vi "Twitter Open.vi"(4 "Access Token Secret (In)":string, 6 "Access Token (In)":string, 8 "error in":errorcluster, 10 "Consumer Secret":string, 11 "Consumer Key":string) -> (0 "error out":errorcluster, 1 "Access Token Secret (Out)":string, 2 "Access Token (Out)":string, 3 "Twitter Handle Out":T1={"OAuth Credentials"={"Signature Method"=enum."HMAC-SHA1", "Version"="1.0", "Client"={"Token"="", "Secret"=""}, "Access"={"Token"="", "Secret"=""}}, "since ID"="", "max ID"="", "Screen Name"=""})   [LabVIEW 2011, in "i3-twitter.lvlib"]
uses:
  i3-twitter.lvlib
  Controls/Twitter Handle.ctl
  i3-oauth/Controls/OAuth Handle.ctl
  i3-oauth/Controls/Signature Method.ctl
  i3-oauth/Controls/Credentials.ctl
  i3-oauth/Controls/Authorization URLs.ctl
  i3-oauth/i3-oauth.lvlib
panel:
  out "Response Header":string
  out "Response Body":string
  # "Debug Only"
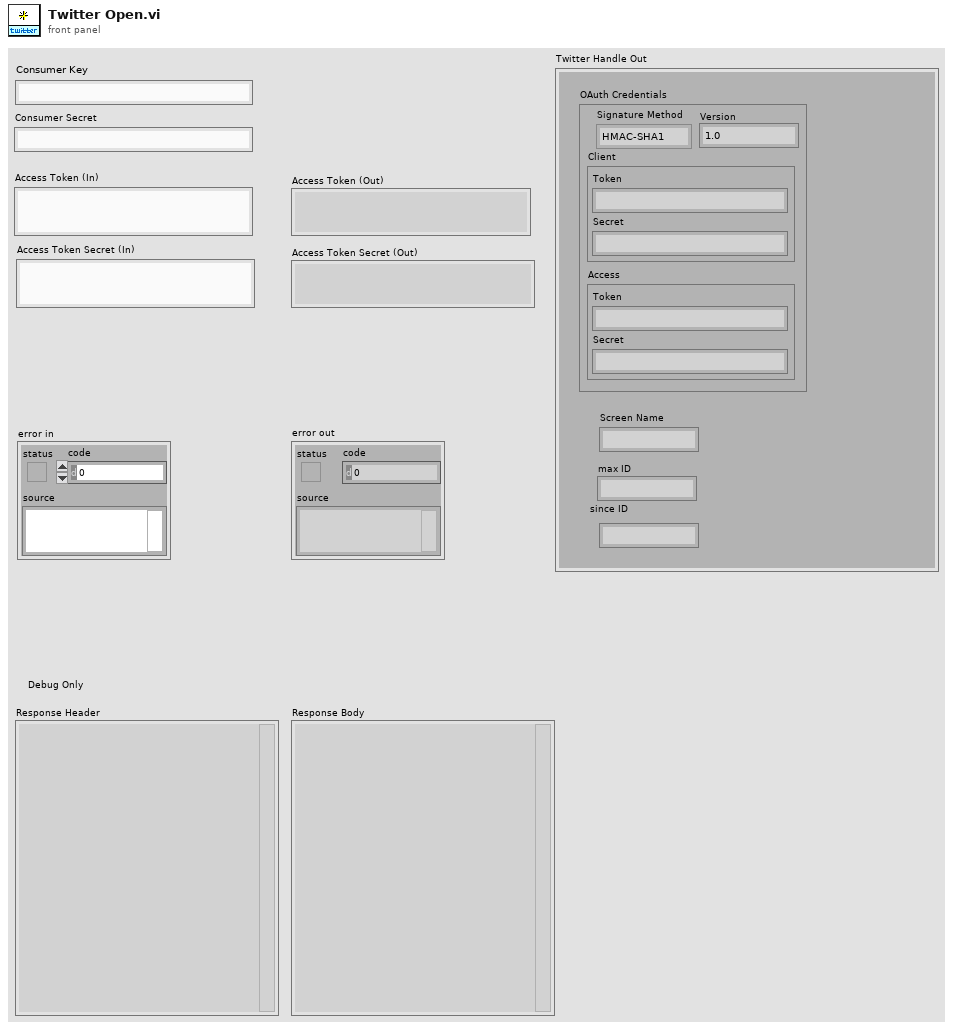
[diagram p1: front panel]
types:
  T1 = typedef "i3-twitter.lvlib/Twitter Handle.ctl" = cluster{"OAuth Credentials":T2, "since ID":string, "max ID":string, "Screen Name":string}
  T2 = typedef "i3-oauth.lvlib/OAuth Handle.ctl" = cluster{"Signature Method":T3, "Version":string, "Client":T4, "Access":T4}
  T3 = typedef "i3-oauth.lvlib/Signature Method.ctl" = enum16{"HMAC-MD5", "HMAC-SHA1", "HMAC-SHA224", "HMAC-SHA256", "HMAC-SHA384", "HMAC-SHA512"}
  T4 = typedef "i3-oauth.lvlib/Credentials.ctl" = cluster{"Token":string, "Secret":string}
  T5 = typedef "i3-oauth.lvlib/Authorization URLs.ctl" = cluster{"Request URL":string, "Authorize URL":string, "Access URL":string}
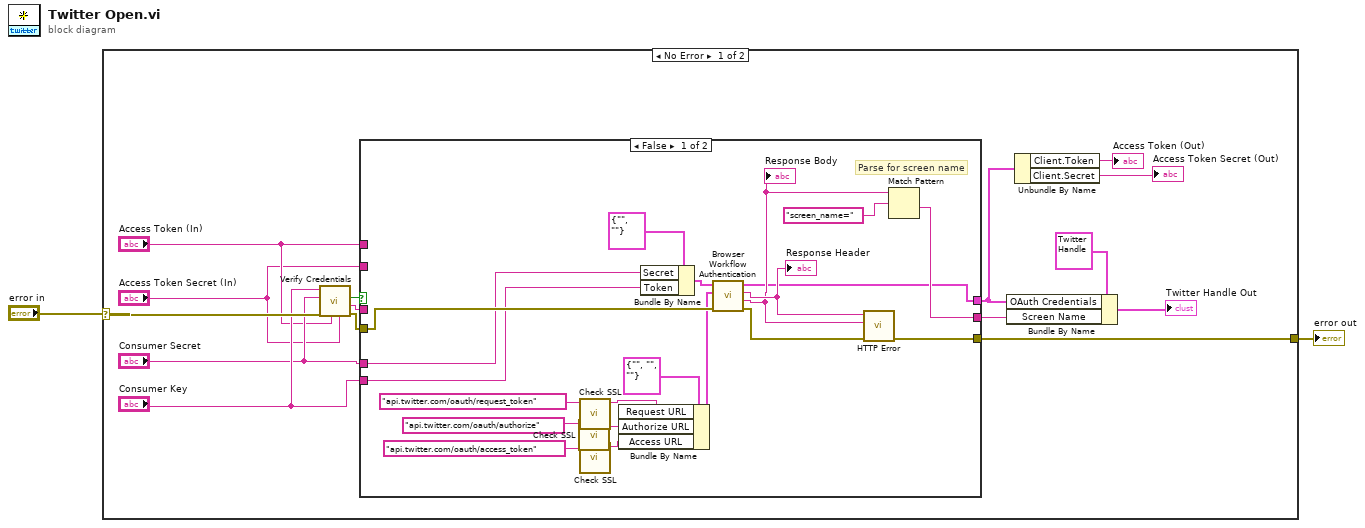
[diagram p0: block diagram]
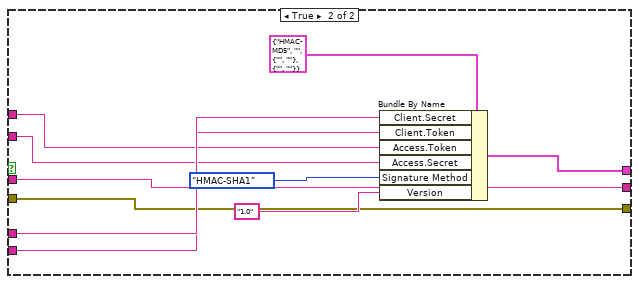
[diagram p2: hidden frame]
diagram:
  n1 = case shown="No Error" "error in" {
    selector: "error in" -> [w7 w48]
    tunnel: [w16 w48] -> w2
    frame No Error {
      n2 = call "Verify Credentials.vi"("Access Token Secret (In)"="Access Token Secret (In)", "Access Token (In)"="Access Token (In)", "error in (no error)"=w7, "Consumer Secret"="Consumer Secret", "Consumer Key"="Consumer Key") -> ("error out"=w13:errorcluster, "Screen Name"=w12:string, "Success?"=w17:bool)  [unwired: 3 in, 1 out]
      n3 = case shown="False" w17 {
        tunnel: "Consumer Secret" -> [w19 w47]
        tunnel: "Consumer Key" -> [w18 w46]
        tunnel: "Access Token (In)" -> [_ w45]
        tunnel: "Access Token Secret (In)" -> [_ w44]
        tunnel: [w28 w41] -> w11
        tunnel: [w35 w39] -> w16
        tunnel: [w37 w38] -> w14
        tunnel: w13 -> [w27 w39]
        tunnel: w12 -> [_ w38]
        frame False {
          # "Parse for screen name"
          n4 = call "Check SSL.vi"("Input URL"="api.twitter.com/oauth/authorize" ("Authorize URL")) -> ("Output URL"=w24:string)  [unwired: 8 in]
          n5 = call "Check SSL.vi"("Input URL"="api.twitter.com/oauth/request_token" ("Request URL")) -> ("Output URL"=w25:string)  [unwired: 8 in]
          n6 = call "Check SSL.vi"("Input URL"="api.twitter.com/oauth/access_token" ("Access URL")) -> ("Output URL"=w23:string)  [unwired: 8 in]
          n7 = Bundle By Name(cluster=T5 {"Request URL"="", "Authorize URL"="", "Access URL"=""} ("Authorization URLs"), "Request URL"=w25, "Authorize URL"=w24, "Access URL"=w23) -> (w22:T5)
          n8 = Bundle By Name(cluster=T4 {"Token"="", "Secret"=""} ("Client Credentials"), "Secret"=w19, "Token"=w18) -> (w21:T4)
          n9 = call "Browser Workflow Authentication.vi"("error in (no error)"=w27, "Authorization URLs"=w22, "Client Credentials"=w21) -> ("error out"=w36:errorcluster, "Access Response Body"=w29:string, "Access Response Header"=w30:string, "OAuth Handle"=w28:T2)  [unwired: 5 in]
          "Response Body" <- w29
          "Response Header" <- w30
          n10 = call "HTTP Error.vi"("error in (no error)"=w36, "Body"=w29, "Header"=w30) -> ("error out"=w35:errorcluster)  [unwired: 6 in, 2 out]
          n11 = Match Pattern(string=w29, regular expression="screen_name=" ("format string")) -> (after substring=w37:string)  [unwired: 1 in, 3 out]
        }
        frame True {
          n12 = Bundle By Name(cluster=T2 {"Signature Method"=enum."HMAC-MD5", "Version"="", "Client"={"Token"="", "Secret"=""}, "Access"={"Token"="", "Secret"=""}} ("OAuth Credentials"), "Client.Secret"=w47, "Client.Token"=w46, "Access.Token"=w45, "Access.Secret"=w44, "Signature Method"=Signature_Method."HMAC-SHA1", "Version"="1.0") -> (w41:T2)
        }
      }
      n13 = Bundle By Name(cluster=T1 {"OAuth Credentials"={"Signature Method"=enum."HMAC-MD5", "Version"="", "Client"={"Token"="", "Secret"=""}, "Access"={"Token"="", "Secret"=""}}, "since ID"="", "max ID"="", "Screen Name"=""} ("Twitter Handle"), "OAuth Credentials"=w11, "Screen Name"=w14) -> (→"Twitter Handle Out":T1)
      n14 = Unbundle By Name(w11) -> ("Client.Token"=→"Access Token (Out)":string, "Client.Secret"=→"Access Token Secret (Out)":string)
    }
    frame Error {
    }
  }
  "error out" <- w2
